vi "AnalogToDigitalConvertor.vi"(0 "Analog_Data(V)":dbl, 5 "Voltage_Range(V)":dbl, 7 "Resolution(bits)":dbl) -> (4 "Digital_Output":dbl)   [LabVIEW 2020]
doc: "This VI gets analog value , range and resolution as inputs and converts it into digital output"
panel:
  # "Analog To Digital Convertor"
  # "This program gets analog data , voltage range and resolution\nand converts it to digital output"
  # "OUTPUT"
  # "INPUT"
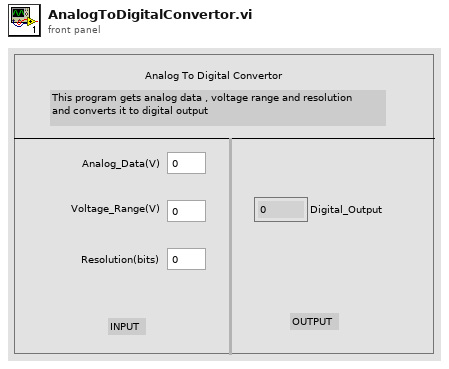
[diagram p1: front panel]
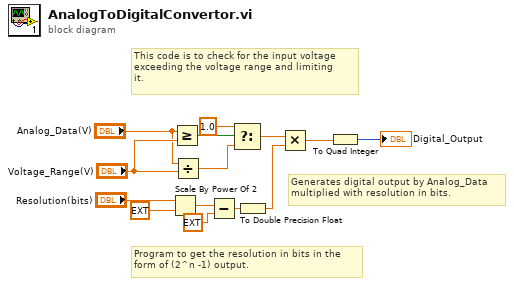
[diagram p0: block diagram]
diagram:
  # "Generates digital output by Analog_Data\nmultiplied with resolution in bits."
  # "Program to get the resolution in bits in the \nform of (2^n -1) output."
  # "This code is to check for the input voltage \nexceeding the voltage range and limiting \nit."
  n1 = Scale By Power Of 2(n="Resolution(bits)", x=ext 1.0) -> (x*2^n=w6:ext)
  n2 = Greater Or Equal?(x="Analog_Data(V)", y="Voltage_Range(V)") -> (x >= y?=w12:bool)
  n3 = Divide(x="Analog_Data(V)", y="Voltage_Range(V)") -> (x/y=w8:dbl)
  n4 = Subtract(x=w6, y=ext 1.0) -> (x-y=w2:ext)
  n5 = Select(t=1.0, s=w12, f=w8) -> (s? t:f=w7:dbl)
  n6 = To Double Precision Float(number=w2) -> (double precision float=w1:dbl)
  n7 = Multiply(x=w7, y=w1) -> (x*y=w4:dbl)
  n8 = To Quad Integer(1:w4) -> (0:→"Digital_Output":i64)
